vi "SV Signal (Waveform).vi"(0 "signal configuration":refnum<class "SV Signal.lvclass">, 1 "reset":bool, 9 "samples":i32=-1, 11 "error in (no error)":errorcluster, 12 "stop":bool) -> (4 "signal configuration":refnum<class "SV Signal.lvclass">, 6 "output waveform":waveform(dbl), 8 "output waveform state":T1=enum."Pre-Measurement Settling", 10 "samples":i32, 14 "done":bool, 15 "error out":errorcluster)   [LabVIEW 2017, in "SV Signal.lvclass"]
doc: "Generates a signal configured by the SV Configure Generator VI and SV Signal Property Nodes. When used in a loop, use a shift register to pass configuration and state contained in <B>signal configuration</B> from one iteration to the next."
uses:
  <vilib>/addons/_NISVFA/_Generation/Signal Generation/SV Signal/SV Signal.lvclass
  <vilib>/addons/_NISVFA/_Generation/Signal Generation/SV Signal/sv_Generation State.ctl
  <vilib>/addons/_NISVFA/_Generation/Signal Generation/SV Signal/sv_System Timing Model.ctl
  <vilib>/addons/_NISVFA/_Generation/Signal Generation/SV Signal/SV Signal.lvclass/SV Signal.ctl
  <vilib>/addons/_NISVFA/_Generation/Signal Generation/SV Continuous Sweep/SV Continuous Sweep.lvclass
  <vilib>/addons/_NISVFA/_Generation/Signal Generation/SV Discrete Sweep/SV Discrete Sweep.lvclass
  <vilib>/addons/_NISVFA/_Generation/Signal Generation/SV Function/SV Function.lvclass
  <vilib>/addons/_NISVFA/_Generation/Signal Generation/SV MLS/SV MLS.lvclass
  <vilib>/addons/_NISVFA/_Generation/Signal Generation/SV Multitone/SV Multitone.lvclass
  <vilib>/addons/_NISVFA/_Generation/Signal Generation/SV Noise/SV Noise.lvclass
  <vilib>/addons/_NISVFA/_Generation/Signal Generation/SV Sinusoid/SV Sinusoid.lvclass
  <vilib>/addons/_NISVFA/_Generation/Signal Generation/SV Square/SV Square.lvclass
  <vilib>/addons/_NISVFA/_Generation/Signal Generation/SV Triangle/SV Triangle.lvclass
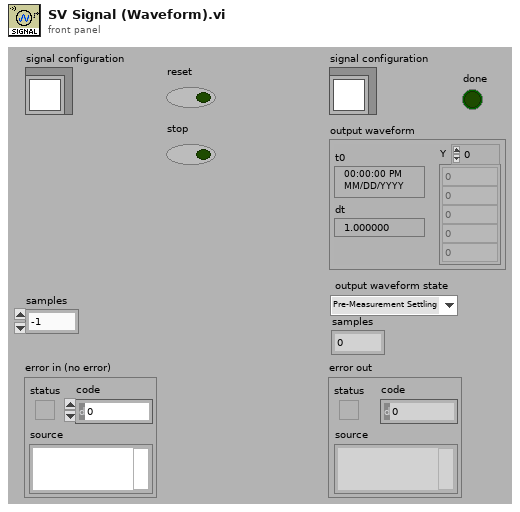
[diagram p1: front panel]
types:
  T1 = typedef "SV Signal.lvclass/sv_Generation State.ctl" = enum16{"Idle", "Ramp Up", "Pre-Measurement Settling", "Measurement", "Post-Measurement Settling", "Discrete Sweep Transition", "Ramp Down", "Update"}
  T2 = typedef "SV Signal.lvclass/sv_System Timing Model.ctl" = i64
  T3 = cluster{"system timing model":T2, "state":cluster{"RESET":bool, "generator timestamp":timestamp, "elapsed seconds":dbl, "elapsed samples":u64, "generation state":T1, "time offset at state":dbl, "samples generated at state":u64, "signal state":variant}, "duration of state":dbl, "samples remaining at state":i32}
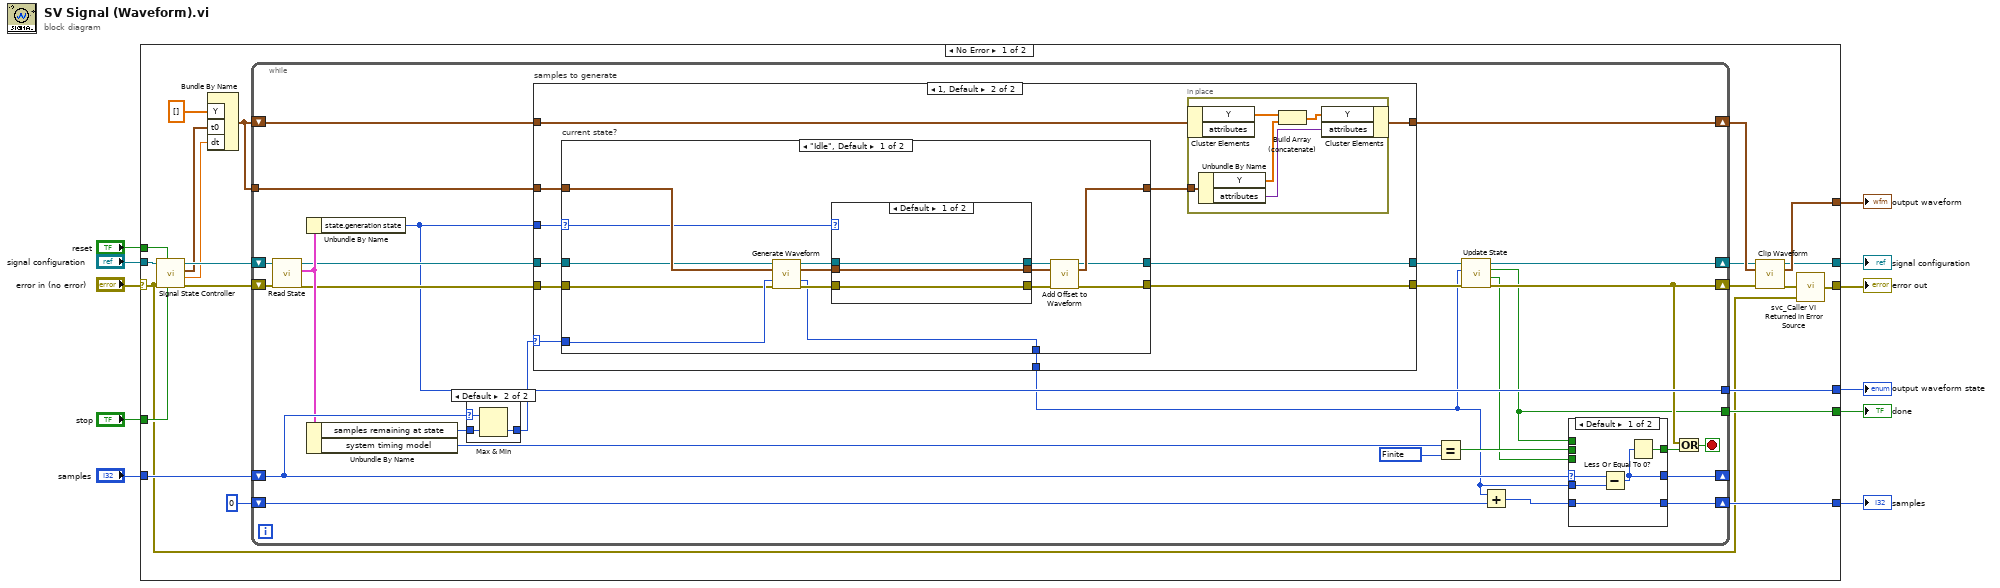
[diagram p0: block diagram]
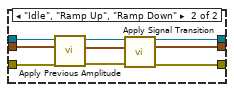
[diagram p3: hidden frame]
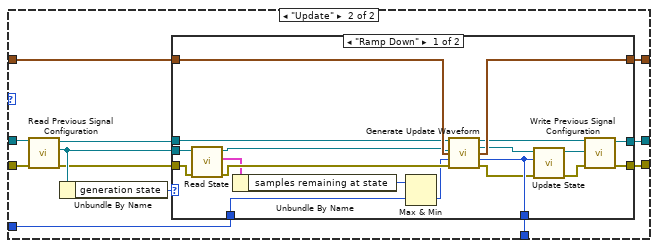
[diagram p4: hidden frame]
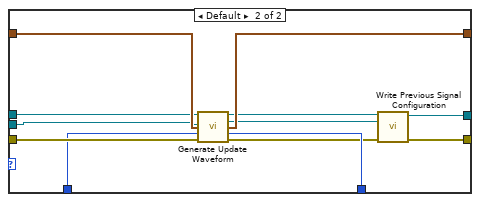
[diagram p5: hidden frame]
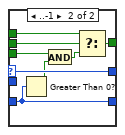
[diagram p6: hidden frame]
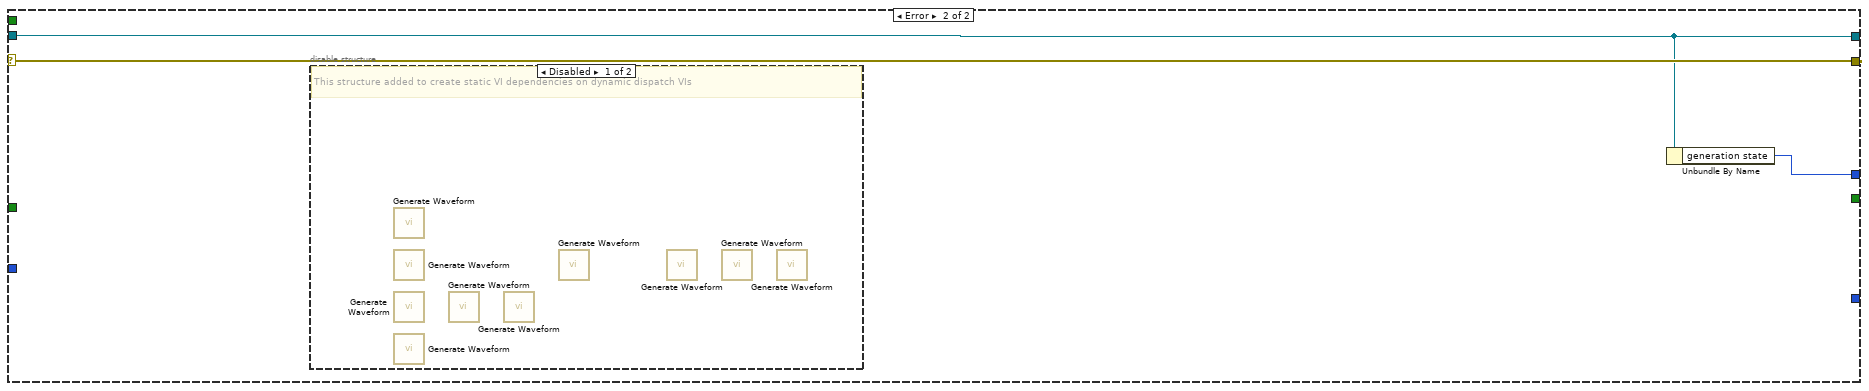
[diagram p8: hidden frame]
diagram:
  n1 = case shown="No Error" "error in (no error)" {
    selector: "error in (no error)" -> [w12 w171]
    tunnel: [w13 w171] -> w10
    tunnel: [w24 w170] -> w8
    tunnel: "signal configuration" -> [w27 w170]
    tunnel: [w25 _] -> w7
    tunnel: [w29 _] -> w6
    tunnel: "reset" -> [w26 _]
    tunnel: "samples" -> [w33 _]
    tunnel: [w28 _] -> w3
    tunnel: "stop" -> [w16 _]
    tunnel: [w15 w169] -> w1
    frame No Error {
      n2 = call <vilib>:"Signal State Controller.vi"("stop"=w16, "reset"=w26, "error IO"=w12, "signal configuration"=w27) -> ("error out"=w31:errorcluster, "waveform dt"=w22:dbl, "waveform t0"=w23:timestamp, "signal configuration"=w30:refnum<class "SV Signal.lvclass">)  [unwired: 4 in]
      n3 = Bundle By Name("Y"=dbl[] [], "t0"=w23, "dt"=w22) -> (w20:waveform(dbl))  [unwired: 1 in]
      n4 = while {
        shift-right: [w40] -> w18
        shift-left: w30 -> [w59]
        shift-right: [w47] -> w29
        shift-left: 0 ("samples") -> [w61]
        shift-right: [w39] -> w17
        shift-left: w31 -> [w58]
        shift-right: [w34] -> w19
        shift-left: w20 -> [w35]
        tunnel: [w38] -> w28
        shift-right: [w53] -> _
        shift-left: w33 -> [w55]
        tunnel: w20 -> [w51]
        tunnel: [w43] -> w15
        stop <- w50 stop-if-true
        w57 = T2 10178 items=["Finite"=10178, "-"=-1, "Continuous"=10123, "-"=-2, "Settled"=110123, "Averaged"=210123, "Discrete Sweep"=310123, "Continuous Sweep"=410123] ("system timing model")
        n5 = call <vilib>:"Read State.vi"("error in (no error)"=w58, "signal configuration"=w59) -> ("error out"=w44:errorcluster, "generator state"=w46:T3, "signal configuration"=w45:refnum<class "SV Signal.lvclass">)  [unwired: 7 in]
        n6 = Unbundle By Name(w46) -> ("state.generation state"=w43:T1)
        n7 = Unbundle By Name(w46) -> ("samples remaining at state"=w52:i32, "system timing model"=w56:T2)
        n8 = case shown="Default" w55 {
          selector: w55 -> [_ w166]
          tunnel: w52 -> [w165 w168]
          tunnel: [w165 w167] -> w60
          frame ..-1 {
          }
          frame Default {
            n9 = Max & Min(x=w166, y=w168) -> (min(x,y)=w167:i32)  [unwired: 1 out]
          }
        }
        n10 = case "samples to generate" shown="1, Default" w60 {
          selector: w60 -> [w64 w76]
          tunnel: w51 -> [_ w75]
          tunnel: w45 -> [w62 w74]
          tunnel: w44 -> [w65 w73]
          tunnel: w43 -> [_ w72]
          tunnel: [w62 w71] -> w42
          tunnel: [w65 w70] -> w41
          tunnel: [w64 w69] -> w36
          tunnel: [w63 w66] -> w34
          tunnel: w35 -> [w63 w67]
          frame ..0 {
          }
          frame 1, Default {
            n11 = case "current state?" shown="\"Idle\", Default" w72 {
              selector: w72 -> [w83 _]
              tunnel: w76 -> [w96 w112]
              tunnel: w74 -> [w82 w119]
              tunnel: [w87 w109] -> w71
              tunnel: [w85 w117] -> w69
              tunnel: [w88 w116] -> w68
              tunnel: w75 -> [w92 w120]
              tunnel: [w86 w110] -> w70
              tunnel: w73 -> [w84 w118]
              frame "Idle", Default {
                n12 = call-dynamic "Generate Waveform.vi"("signal configuration and state in"=w82, "template waveform"=w92, "samples"=w96, "error in (no error)"=w84) -> ("signal configuration and state out"=w95:refnum<class "SV Signal.lvclass">, "output waveform"=w93:waveform(dbl), "samples"=w85:i32, "error out"=w94:errorcluster)  [unwired: 8 in]
                n13 = case shown="Default" w83 {
                  tunnel: w95 -> [w99 w105]
                  tunnel: w94 -> [w97 w101]
                  tunnel: w93 -> [w98 w103]
                  tunnel: [w99 w108] -> w91
                  tunnel: [w98 w107] -> w90
                  tunnel: [w97 w106] -> w89
                  frame Default {
                  }
                  frame "Idle", "Ramp Up", "Ramp Down" {
                    n14 = call <vilib>:"Apply Previous Amplitude.vi"("error in (no error)"=w101, "waveform in"=w103, "SV Signal in"=w105) -> ("error out"=w100:errorcluster, "waveform out"=w102:waveform(dbl), "SV Signal out"=w104:refnum<class "SV Signal.lvclass">)  [unwired: 6 in]
                    n15 = call <vilib>:"Apply Signal Transition.vi"("signal configuration and state in"=w104, "waveform"=w102, "error in (no error)"=w100) -> ("signal configuration and state out"=w108:refnum<class "SV Signal.lvclass">, "profiled waveform"=w107:waveform(dbl), "error out"=w106:errorcluster)  [unwired: 10 in]
                  }
                }
                n16 = call <vilib>:"Add Offset to Waveform.vi"("signal configuration"=w91, "input waveform"=w90, "error in (no error)"=w89) -> ("signal configuration"=w87:refnum<class "SV Signal.lvclass">, "offset waveform"=w88:waveform(dbl), "error out"=w86:errorcluster)  [unwired: 9 in, 1 out]
              }
              frame "Update" {
                n17 = call <vilib>:"Read Previous Signal Configuration.vi"("error in (no error)"=w118, "current signal configuration in"=w119) -> ("error out"=w113:errorcluster, "previous signal configuration"=w114:refnum<class "SV Signal.lvclass">, "current signal configuration out"=w115:refnum<class "SV Signal.lvclass">)  [unwired: 7 in]
                n18 = Unbundle By Name(w114) -> ("generation state"=w111:T1)
                n19 = case shown="\"Ramp Down\"" w111 {
                  tunnel: w120 -> [w139 w151]
                  tunnel: [w138 w150] -> w109
                  tunnel: [w137 w149] -> w110
                  tunnel: [w136 w148] -> w117
                  tunnel: [w135 w147] -> w116
                  tunnel: w115 -> [w134 w146]
                  tunnel: w114 -> [w132 w143]
                  tunnel: w113 -> [w130 w142]
                  tunnel: w112 -> [w129 w141]
                  frame "Ramp Down" {
                    n20 = call <vilib>:"Read State.vi"("error in (no error)"=w130, "signal configuration"=w132) -> ("error out"=w131:errorcluster, "generator state"=w127:T3, "signal configuration"=w133:refnum<class "SV Signal.lvclass">)  [unwired: 7 in]
                    n21 = Unbundle By Name(w127) -> ("samples remaining at state"=w126:i32)
                    n22 = Max & Min(x=w126, y=w129) -> (min(x,y)=w128:i32)  [unwired: 1 out]
                    n23 = call-dynamic "Generate Update Waveform.vi"("updated signal in"=w134, "previous signal"=w133, "template waveform"=w139, "samples"=w128, "error in (no error)"=w131) -> ("updated signal out"=w123:refnum<class "SV Signal.lvclass">, "previous signal out"=w122:refnum<class "SV Signal.lvclass">, "output waveform"=w135:waveform(dbl), "samples generated"=w136:i32, "error out"=w121:errorcluster)  [unwired: 6 in]
                    n24 = call-dynamic "Update State.vi"("error in (no error)"=w121, "samples generated"=w136, "signal configuration"=w122) -> ("error out"=w125:errorcluster, "signal configuration"=w124:refnum<class "SV Signal.lvclass">)  [unwired: 4 in, 3 out]
                    n25 = call <vilib>:"Write Previous Signal Configuration.vi"("error in (no error)"=w125, "previous signal configuration"=w124, "current signal configuration in"=w123) -> ("error out"=w137:errorcluster, "current signal configuration out"=w138:refnum<class "SV Signal.lvclass">)  [unwired: 7 in]
                  }
                  frame Default {
                    n26 = call-dynamic "Generate Update Waveform.vi"("updated signal in"=w146, "previous signal"=w143, "template waveform"=w151, "samples"=w141, "error in (no error)"=w142) -> ("updated signal out"=w144:refnum<class "SV Signal.lvclass">, "previous signal out"=w140:refnum<class "SV Signal.lvclass">, "output waveform"=w147:waveform(dbl), "samples generated"=w148:i32, "error out"=w145:errorcluster)  [unwired: 6 in]
                    n27 = call <vilib>:"Write Previous Signal Configuration.vi"("error in (no error)"=w145, "previous signal configuration"=w140, "current signal configuration in"=w144) -> ("error out"=w149:errorcluster, "current signal configuration out"=w150:refnum<class "SV Signal.lvclass">)  [unwired: 7 in]
                  }
                }
              }
            }
            n28 = in-place {
              in-place-border: w68 -> [w80]
              n29 = in-place-cluster #1(w67) -> ("Y"=w79:dbl[])  [unwired: 1 out]
              n30 = Unbundle By Name(w80) -> ("Y"=w81:dbl[], "attributes"=w77:variant)
              n31 = Build Array (concatenate)(w79, w81) -> (w78:dbl[])
              n32 = in-place-cluster #1("Y"=w78, "attributes"=w77) -> (w66:waveform(dbl))
            }
          }
        }
        n33 = Equal?(x=w56, y=w57) -> (x = y?=w54:bool)
        n34 = call-dynamic "Update State.vi"("error in (no error)"=w41, "samples generated"=w36, "signal configuration"=w42) -> ("error out"=w39:errorcluster, "segment done"=w37:bool, "generation done"=w38:bool, "signal configuration"=w40:refnum<class "SV Signal.lvclass">)  [unwired: 4 in, 1 out]
        n35 = Add(x=w36, y=w61) -> (x+y=w48:i32)
        n36 = case shown="Default" w55 {
          selector: w55 -> [w155 w161]
          tunnel: w54 -> [_ w164]
          tunnel: w37 -> [_ w160]
          tunnel: w38 -> [_ w163]
          tunnel: [w154 w162] -> w49
          tunnel: [w153 w161] -> w53
          tunnel: w36 -> [w156 _]
          tunnel: w48 -> [w152 w159]
          tunnel: [w152 w159] -> w47
          frame Default {
            n37 = Subtract(x=w155, y=w156) -> (x-y=w153:i32)
            n38 = Less Or Equal To 0?(x=w153) -> (x <= 0?=w154:bool)
          }
          frame ..-1 {
            n39 = Greater Than 0?(x=w159) -> (x > 0?=w158:bool)
            n40 = And(x=w160, y=w158) -> (x .and. y?=w157:bool)
            n41 = Select(t=w163, s=w164, f=w157) -> (s? t:f=w162:bool)
          }
        }
        n42 = Or(x=w39, y=w49) -> (x .or. y?=w50:bool)
      }
      n43 = call <vilib>:"Clip Waveform.vi"("signal configuration"=w18, "input waveform"=w19, "error in (no error)"=w17) -> ("signal configuration"=w24:refnum<class "SV Signal.lvclass">, "offset waveform"=w25:waveform(dbl), "error out"=w14:errorcluster)  [unwired: 10 in]
      n44 = call <vilib>:"svc_Caller VI Returned in Error Source.vi"("warning input to caller"=w12, "error in (no error)"=w14) -> ("error out"=w13:errorcluster)  [unwired: 3 in]
    }
    frame Error {
      n45 = disable-structure shown="Disabled" {
        frame Disabled {
          # "This structure added to create static VI dependencies on dynamic dispatch VIs"
          n46 = call-dynamic "Generate Waveform.vi"() -> ()  [unwired: 12 in, 4 out]
          n47 = call-dynamic "Generate Waveform.vi"() -> ()  [unwired: 12 in, 4 out]
          n48 = call-dynamic "Generate Waveform.vi"() -> ()  [unwired: 12 in, 4 out]
          n49 = call-dynamic "Generate Waveform.vi"() -> ()  [unwired: 12 in, 4 out]
          n50 = call-dynamic "Generate Waveform.vi"() -> ()  [unwired: 12 in, 4 out]
          n51 = call-dynamic "Generate Waveform.vi"() -> ()  [unwired: 12 in, 4 out]
          n52 = call-dynamic "Generate Waveform.vi"() -> ()  [unwired: 12 in, 4 out]
          n53 = call-dynamic "Generate Waveform.vi"() -> ()  [unwired: 12 in, 4 out]
          n54 = call-dynamic "Generate Waveform.vi"() -> ()  [unwired: 12 in, 4 out]
          n55 = call-dynamic "Generate Waveform.vi"() -> ()  [unwired: 12 in, 4 out]
        }
        frame Enabled {
        }
      }
      n56 = Unbundle By Name(w170) -> ("generation state"=w169:T1)
    }
  }
  "error out" <- w10
  "signal configuration" <- w8
  "output waveform" <- w7
  "samples" <- w6
  "done" <- w3
  "output waveform state" <- w1
